vi "Lab Panel V5.12.vi"() -> ()   [LabVIEW 2013] (continued)
                            n1494 = local write "DISP LAB05-2"(w2801) -> ()
                          }
                        }
                      }
                      frame False {
                      }
                    }
                  }
                }
              }
            }
          }
          frame #6 {
            # "end test & close test files"
            n1495 = local read "MAIL SETTINGS"() -> (w2807:T7)
            n1496 = Unbundle(w2807) -> ("OUT SERVER ADDRESS"=w2806:string, "FROM ACCOUNT"=w2805:string)  [unwired: 5 out]
            n1497 = stacked-sequence {
              tunnel: w2817 -> [_ _ _ _ _ _ _ _ _ _]
              tunnel: w2818 -> [_ _ _ _ _ _ _ _ _ _]
              tunnel: w2816 -> [_ _ _ _ _ _ _ _ _ _]
              tunnel: w2815 -> [_ _ _ _ _ _ _ _ _ _]
              tunnel: w2814 -> [_ _ _ _ _ _ _ _ _ _]
              tunnel: w2813 -> [_ _ _ _ _ _ _ _ _ _]
              tunnel: w2812 -> [_ _ _ _ _ _ _ _ _ _]
              tunnel: w2811 -> [_ _ _ _ _ _ _ _ _ _]
              tunnel: w2810 -> [_ _ _ _ _ _ _ _ _ _]
              tunnel: w2809 -> [_ _ _ _ _ _ _ _ _ _]
              tunnel: w2806 -> [w2822 w2874 w2922 w2969 w3016 w3063 w3110 w3157 w3204 w3251]
              tunnel: w2805 -> [w2821 w2873 w2921 w2968 w3015 w3062 w3109 w3156 w3203 w3250]
              tunnel: "Mail Test File To:" -> [w2820 w2872 w2920 w2967 w3014 w3061 w3108 w3155 w3202 w3249]
              tunnel: "Mail Test Fail" -> [w2819 w2871 w2919 w2966 w3013 w3060 w3107 w3154 w3201 w3248]
              frame #0 {
                # "LAB01-1"
                n1498 = local read "DISP LAB01-1"() -> (w2826:T4)
                n1499 = local read "run lab01-1"() -> (w2823:bool)
                n1500 = local read "TDMS LAB01-1"() -> (w2824:refnum<k34>)
                n1501 = Unbundle(w2826) -> ("CYCLE"=w2827:dbl, "STATUS"=w2825:string)  [unwired: 1 out]
                n1502 = case shown="True" w2823 {
                  tunnel: w2827 -> [_ w2833]
                  tunnel: w2826 -> [_ w2835]
                  tunnel: w2825 -> [_ w2832]
                  tunnel: w2824 -> [_ w2834]
                  tunnel: w2822 -> [_ w2831]
                  tunnel: w2821 -> [_ w2830]
                  tunnel: w2820 -> [_ w2829]
                  tunnel: w2819 -> [_ w2828]
                  frame False {
                  }
                  frame True {
                    n1503 = Not Equal?(x=w2832, y="RUN") -> (x != y?=w2836:bool)
                    n1504 = Greater?(x=w2833, y=2.0) -> (0:w2838:bool)
                    n1505 = And(x=w2838, y=w2836) -> (x .and. y?=w2837:bool)
                    n1506 = case shown="True" w2837 {
                      tunnel: w2835 -> [_ w2848]
                      tunnel: w2834 -> [_ w2847]
                      tunnel: w2833 -> [_ w2846]
                      tunnel: w2832 -> [_ w2845]
                      tunnel: w2831 -> [_ w2844]
                      tunnel: w2830 -> [_ w2843]
                      tunnel: w2829 -> [_ w2842]
                      tunnel: w2828 -> [_ w2841]
                      frame False {
                      }
                      frame True {
                        n1507 = stacked-sequence {
                          tunnel: w2848 -> [w2852 _ _]
                          tunnel: w2847 -> [_ w2854 _]
                          tunnel: w2846 -> [_ _ _]
                          tunnel: w2845 -> [_ _ w2860]
                          tunnel: w2844 -> [_ _ w2859]
                          tunnel: w2843 -> [_ _ w2858]
                          tunnel: w2842 -> [_ _ w2857]
                          tunnel: w2841 -> [_ _ w2856]
                          frame #0 {
                            w2849 = FALSE
                            n1508 = local write "mail control"("END") -> ()
                            n1509 = Bundle(cluster=w2852) -> (w2851:T4)  [unwired: 3 in]
                            n1510 = local write "DISP LAB01-1"(w2851) -> ()
                            n1511 = local write "O/I  LAB01-1"(w2849) -> ()
                            n1512 = local write "run lab01-1"(w2849) -> ()
                            n1513 = local write "RUN LAB01-1"(w2849) -> ()
                          }
                          frame #1 {
                            n1514 = TDMS Close(11:w2854) -> (0:w2853:errorcluster)  [unwired: 1 in, 1 out]
                            n1515 = local write "data file error"(w2853) -> ()
                          }
                          frame #2 {
                            n1516 = stacked-sequence {
                              tunnel: "LAB01-1" -> [w2862 w2864 _]
                              tunnel: w2860 -> [_ w2870 _]
                              tunnel: w2859 -> [_ w2869 _]
                              tunnel: w2858 -> [_ w2868 _]
                              tunnel: w2857 -> [_ w2867 _]
                              tunnel: w2856 -> [_ w2866 _]
                              frame #0 {
                                n1517 = call "sub vi - defrag tdms v1.vi"("panel id"=w2862) -> ("error out"=w2861:errorcluster)  [unwired: 10 in]
                                n1518 = local write "data file error"(w2861) -> ()
                              }
                              frame #1 {
                                n1519 = Bundle("STATUS"=w2870, "OUT SERVER ADDRESS"=w2869, "FROM ACCOUNT"=w2868, "Mail Test File To:"=w2867, "Mail Test Fail"=w2866) -> (w2863:T25)  [unwired: 1 in]
                                n1520 = call "Save data file (pass-fail) v5.vi"("Input Cluster"=w2863, "panel id"=w2864) -> ("network file save error"=w2865:errorcluster)  [unwired: 8 in, 1 out]
                                n1521 = local write "data file error"(w2865) -> ()
                              }
                              frame #2 {
                              }
                            }
                          }
                        }
                      }
                    }
                  }
                }
              }
              frame #1 {
                # "LAB01-2"
                n1522 = local read "run lab01-2"() -> (w2875:bool)
                n1523 = case shown="True" w2875 {
                  tunnel: w2874 -> [_ w2879]
                  tunnel: w2873 -> [_ w2878]
                  tunnel: w2872 -> [_ w2877]
                  tunnel: w2871 -> [_ w2876]
                  frame False {
                  }
                  frame True {
                    n1524 = local read "DISP LAB01-2"() -> (w2887:T4)
                    n1525 = local read "TDMS LAB01-2"() -> (w2886:refnum<k34>)
                    n1526 = Unbundle(w2887) -> ("CYCLE"=w2881:dbl, "STATUS"=w2880:string)  [unwired: 1 out]
                    n1527 = Not Equal?(x=w2880, y="RUN") -> (x != y?=w2883:bool)
                    n1528 = Greater?(x=w2881, y=2.0) -> (0:w2884:bool)
                    n1529 = And(x=w2884, y=w2883) -> (x .and. y?=w2882:bool)
                    n1530 = case shown="True" w2882 {
                      tunnel: w2887 -> [_ w2896]
                      tunnel: w2886 -> [_ w2895]
                      tunnel: w2881 -> [_ w2894]
                      tunnel: w2880 -> [_ w2893]
                      tunnel: w2879 -> [_ w2892]
                      tunnel: w2878 -> [_ w2891]
                      tunnel: w2877 -> [_ w2890]
                      tunnel: w2876 -> [_ w2889]
                      frame False {
                      }
                      frame True {
                        n1531 = stacked-sequence {
                          tunnel: w2896 -> [w2899 _ _]
                          tunnel: w2895 -> [_ w2901 _]
                          tunnel: w2894 -> [_ _ _]
                          tunnel: w2893 -> [_ _ w2907]
                          tunnel: w2892 -> [_ _ w2906]
                          tunnel: w2891 -> [_ _ w2905]
                          tunnel: w2890 -> [_ _ w2904]
                          tunnel: w2889 -> [_ _ w2903]
                          frame #0 {
                            w2897 = FALSE
                            n1532 = local write "mail control"("END") -> ()
                            n1533 = Bundle(cluster=w2899) -> (w2900:T4)  [unwired: 3 in]
                            n1534 = local write "RUN LAB01-2"(w2897) -> ()
                            n1535 = local write "run lab01-2"(w2897) -> ()
                            n1536 = local write "O/I  LAB01-2"(w2897) -> ()
                            n1537 = local write "DISP LAB01-2"(w2900) -> ()
                          }
                          frame #1 {
                            n1538 = TDMS Close(11:w2901) -> (0:w2902:errorcluster)  [unwired: 1 in, 1 out]
                            n1539 = local write "data file error"(w2902) -> ()
                          }
                          frame #2 {
                            n1540 = stacked-sequence {
                              tunnel: "LAB01-2" -> [w2910 w2911]
                              tunnel: w2907 -> [_ w2916]
                              tunnel: w2906 -> [_ w2915]
                              tunnel: w2905 -> [_ w2914]
                              tunnel: w2904 -> [_ w2913]
                              tunnel: w2903 -> [_ w2912]
                              frame #0 {
                                n1541 = call "sub vi - defrag tdms v1.vi"("panel id"=w2910) -> ("error out"=w2909:errorcluster)  [unwired: 10 in]
                                n1542 = local write "data file error"(w2909) -> ()
                              }
                              frame #1 {
                                n1543 = Bundle("STATUS"=w2916, "OUT SERVER ADDRESS"=w2915, "FROM ACCOUNT"=w2914, "Mail Test File To:"=w2913, "Mail Test Fail"=w2912) -> (w2918:T25)  [unwired: 1 in]
                                n1544 = call "Save data file (pass-fail) v5.vi"("Input Cluster"=w2918, "panel id"=w2911) -> ("network file save error"=w2917:errorcluster)  [unwired: 8 in, 1 out]
                                n1545 = local write "data file error"(w2917) -> ()
                              }
                            }
                          }
                        }
                      }
                    }
                  }
                }
              }
              frame #2 {
                # "LAB02-1"
                n1546 = local read "run lab02-1"() -> (w2923:bool)
                n1547 = case shown="True" w2923 {
                  tunnel: w2922 -> [_ w2927]
                  tunnel: w2921 -> [_ w2926]
                  tunnel: w2920 -> [_ w2925]
                  tunnel: w2919 -> [_ w2924]
                  frame False {
                  }
                  frame True {
                    n1548 = local read "DISP LAB02-1"() -> (w2935:T4)
                    n1549 = Unbundle(w2935) -> ("CYCLE"=w2931:dbl, "STATUS"=w2928:string)  [unwired: 1 out]
                    n1550 = local read "TDMS LAB02-1"() -> (w2934:refnum<k34>)
                    n1551 = Not Equal?(x=w2928, y="RUN") -> (x != y?=w2930:bool)
                    n1552 = Greater?(x=w2931, y=2.0) -> (0:w2932:bool)
                    n1553 = And(x=w2932, y=w2930) -> (x .and. y?=w2929:bool)
                    n1554 = case shown="True" w2929 {
                      tunnel: w2935 -> [_ w2943]
                      tunnel: w2934 -> [_ w2942]
                      tunnel: w2928 -> [_ w2941]
                      tunnel: w2927 -> [_ w2940]
                      tunnel: w2926 -> [_ w2939]
                      tunnel: w2925 -> [_ w2938]
                      tunnel: w2924 -> [_ w2937]
                      frame False {
                      }
                      frame True {
                        n1555 = stacked-sequence {
                          tunnel: w2943 -> [w2946 _ _]
                          tunnel: w2942 -> [_ w2948 _]
                          tunnel: w2941 -> [_ _ w2954]
                          tunnel: w2940 -> [_ _ w2953]
                          tunnel: w2939 -> [_ _ w2952]
                          tunnel: w2938 -> [_ _ w2951]
                          tunnel: w2937 -> [_ _ w2950]
                          frame #0 {
                            w2944 = FALSE
                            n1556 = local write "mail control"("END") -> ()
                            n1557 = Bundle(cluster=w2946) -> (w2947:T4)  [unwired: 3 in]
                            n1558 = local write "O/I  LAB02-1"(w2944) -> ()
                            n1559 = local write "RUN LAB02-1"(w2944) -> ()
                            n1560 = local write "run lab02-1"(w2944) -> ()
                            n1561 = local write "DISP LAB02-1"(w2947) -> ()
                          }
                          frame #1 {
                            n1562 = TDMS Close(11:w2948) -> (0:w2949:errorcluster)  [unwired: 1 in, 1 out]
                            n1563 = local write "data file error"(w2949) -> ()
                          }
                          frame #2 {
                            n1564 = stacked-sequence {
                              tunnel: "LAB02-1" -> [w2957 w2964]
                              tunnel: w2954 -> [_ w2962]
                              tunnel: w2953 -> [_ w2961]
                              tunnel: w2952 -> [_ w2960]
                              tunnel: w2951 -> [_ w2959]
                              tunnel: w2950 -> [_ w2958]
                              frame #0 {
                                n1565 = call "sub vi - defrag tdms v1.vi"("panel id"=w2957) -> ("error out"=w2956:errorcluster)  [unwired: 10 in]
                                n1566 = local write "data file error"(w2956) -> ()
                              }
                              frame #1 {
                                n1567 = Bundle("STATUS"=w2962, "OUT SERVER ADDRESS"=w2961, "FROM ACCOUNT"=w2960, "Mail Test File To:"=w2959, "Mail Test Fail"=w2958) -> (w2963:T25)  [unwired: 1 in]
                                n1568 = call "Save data file (pass-fail) v5.vi"("Input Cluster"=w2963, "panel id"=w2964) -> ("network file save error"=w2965:errorcluster)  [unwired: 8 in, 1 out]
                                n1569 = local write "data file error"(w2965) -> ()
                              }
                            }
                          }
                        }
                      }
                    }
                  }
                }
              }
              frame #3 {
                # "LAB02-2"
                n1570 = local read "run lab02-2"() -> (w2970:bool)
                n1571 = case shown="True" w2970 {
                  tunnel: w2969 -> [_ w2974]
                  tunnel: w2968 -> [_ w2973]
                  tunnel: w2967 -> [_ w2972]
                  tunnel: w2966 -> [_ w2971]
                  frame False {
                  }
                  frame True {
                    n1572 = local read "DISP LAB02-2"() -> (w2982:T4)
                    n1573 = local read "TDMS LAB02-2"() -> (w2981:refnum<k34>)
                    n1574 = Unbundle(w2982) -> ("CYCLE"=w2978:dbl, "STATUS"=w2975:string)  [unwired: 1 out]
                    n1575 = Not Equal?(x=w2975, y="RUN") -> (x != y?=w2977:bool)
                    n1576 = Greater?(x=w2978, y=2.0) -> (0:w2979:bool)
                    n1577 = And(x=w2979, y=w2977) -> (x .and. y?=w2976:bool)
                    n1578 = case shown="True" w2976 {
                      tunnel: w2982 -> [_ w2990]
                      tunnel: w2981 -> [_ w2989]
                      tunnel: w2975 -> [_ w2988]
                      tunnel: w2974 -> [_ w2987]
                      tunnel: w2973 -> [_ w2986]
                      tunnel: w2972 -> [_ w2985]
                      tunnel: w2971 -> [_ w2984]
                      frame False {
                      }
                      frame True {
                        n1579 = stacked-sequence {
                          tunnel: w2990 -> [w2993 _ _]
                          tunnel: w2989 -> [_ w2995 _]
                          tunnel: w2988 -> [_ _ w3001]
                          tunnel: w2987 -> [_ _ w3000]
                          tunnel: w2986 -> [_ _ w2999]
                          tunnel: w2985 -> [_ _ w2998]
                          tunnel: w2984 -> [_ _ w2997]
                          frame #0 {
                            w2991 = FALSE
                            n1580 = local write "mail control"("END") -> ()
                            n1581 = Bundle(cluster=w2993) -> (w2994:T4)  [unwired: 3 in]
                            n1582 = local write "O/I  LAB02-2"(w2991) -> ()
                            n1583 = local write "run lab02-2"(w2991) -> ()
                            n1584 = local write "RUN LAB02-2"(w2991) -> ()
                            n1585 = local write "DISP LAB02-2"(w2994) -> ()
                          }
                          frame #1 {
                            n1586 = TDMS Close(11:w2995) -> (0:w2996:errorcluster)  [unwired: 1 in, 1 out]
                            n1587 = local write "data file error"(w2996) -> ()
                          }
                          frame #2 {
                            n1588 = stacked-sequence {
                              tunnel: "LAB02-2" -> [w3004 w3010]
                              tunnel: w3001 -> [_ w3009]
                              tunnel: w3000 -> [_ w3008]
                              tunnel: w2999 -> [_ w3007]
                              tunnel: w2998 -> [_ w3006]
                              tunnel: w2997 -> [_ w3005]
                              frame #0 {
                                n1589 = call "sub vi - defrag tdms v1.vi"("panel id"=w3004) -> ("error out"=w3003:errorcluster)  [unwired: 10 in]
                                n1590 = local write "data file error"(w3003) -> ()
                              }
                              frame #1 {
                                n1591 = Bundle("STATUS"=w3009, "OUT SERVER ADDRESS"=w3008, "FROM ACCOUNT"=w3007, "Mail Test File To:"=w3006, "Mail Test Fail"=w3005) -> (w3012:T25)  [unwired: 1 in]
                                n1592 = call "Save data file (pass-fail) v5.vi"("Input Cluster"=w3012, "panel id"=w3010) -> ("network file save error"=w3011:errorcluster)  [unwired: 8 in, 1 out]
                                n1593 = local write "data file error"(w3011) -> ()
                              }
                            }
                          }
                        }
                      }
                    }
                  }
                }
              }
              frame #4 {
                # "LAB03-1"
                n1594 = local read "run lab03-1"() -> (w3017:bool)
                n1595 = case shown="True" w3017 {
                  tunnel: w3016 -> [_ w3021]
                  tunnel: w3015 -> [_ w3020]
                  tunnel: w3014 -> [_ w3019]
                  tunnel: w3013 -> [_ w3018]
                  frame False {
                  }
                  frame True {
                    n1596 = local read "DISP LAB03-1"() -> (w3029:T4)
                    n1597 = local read "TDMS LAB03-1"() -> (w3028:refnum<k34>)
                    n1598 = Unbundle(w3029) -> ("CYCLE"=w3025:dbl, "STATUS"=w3022:string)  [unwired: 1 out]
                    n1599 = Not Equal?(x=w3022, y="RUN") -> (x != y?=w3024:bool)
                    n1600 = Greater?(x=w3025, y=2.0) -> (0:w3026:bool)
                    n1601 = And(x=w3026, y=w3024) -> (x .and. y?=w3023:bool)
                    n1602 = case shown="True" w3023 {
                      tunnel: w3029 -> [_ w3037]
                      tunnel: w3028 -> [_ w3036]
                      tunnel: w3022 -> [_ w3035]
                      tunnel: w3021 -> [_ w3034]
                      tunnel: w3020 -> [_ w3033]
                      tunnel: w3019 -> [_ w3032]
                      tunnel: w3018 -> [_ w3031]
                      frame False {
                      }
                      frame True {
                        n1603 = stacked-sequence {
                          tunnel: w3037 -> [w3040 _ _]
                          tunnel: w3036 -> [_ w3042 _]
                          tunnel: w3035 -> [_ _ w3048]
                          tunnel: w3034 -> [_ _ w3047]
                          tunnel: w3033 -> [_ _ w3046]
                          tunnel: w3032 -> [_ _ w3045]
                          tunnel: w3031 -> [_ _ w3044]
                          frame #0 {
                            w3038 = FALSE
                            n1604 = local write "mail control"("END") -> ()
                            n1605 = Bundle(cluster=w3040) -> (w3041:T4)  [unwired: 3 in]
                            n1606 = local write "O/I  LAB03-1"(w3038) -> ()
                            n1607 = local write "run lab03-1"(w3038) -> ()
                            n1608 = local write "RUN LAB03-1"(w3038) -> ()
                            n1609 = local write "DISP LAB03-1"(w3041) -> ()
                          }
                          frame #1 {
                            n1610 = TDMS Close(11:w3042) -> (0:w3043:errorcluster)  [unwired: 1 in, 1 out]
                            n1611 = local write "data file error"(w3043) -> ()
                          }
                          frame #2 {
                            n1612 = stacked-sequence {
                              tunnel: "LAB03-1" -> [w3051 w3057]
                              tunnel: w3048 -> [_ w3056]
                              tunnel: w3047 -> [_ w3055]
                              tunnel: w3046 -> [_ w3054]
                              tunnel: w3045 -> [_ w3053]
                              tunnel: w3044 -> [_ w3052]
                              frame #0 {
                                n1613 = call "sub vi - defrag tdms v1.vi"("panel id"=w3051) -> ("error out"=w3050:errorcluster)  [unwired: 10 in]
                                n1614 = local write "data file error"(w3050) -> ()
                              }
                              frame #1 {
                                n1615 = Bundle("STATUS"=w3056, "OUT SERVER ADDRESS"=w3055, "FROM ACCOUNT"=w3054, "Mail Test File To:"=w3053, "Mail Test Fail"=w3052) -> (w3059:T25)  [unwired: 1 in]
                                n1616 = call "Save data file (pass-fail) v5.vi"("Input Cluster"=w3059, "panel id"=w3057) -> ("network file save error"=w3058:errorcluster)  [unwired: 8 in, 1 out]
                                n1617 = local write "data file error"(w3058) -> ()
                              }
                            }
                          }
                        }
                      }
                    }
                  }
                }
              }
              frame #5 {
                # "LAB03-2"
                n1618 = local read "run lab03-2"() -> (w3064:bool)
                n1619 = case shown="True" w3064 {
                  tunnel: w3063 -> [_ w3068]
                  tunnel: w3062 -> [_ w3067]
                  tunnel: w3061 -> [_ w3066]
                  tunnel: w3060 -> [_ w3065]
                  frame False {
                  }
                  frame True {
                    n1620 = local read "DISP LAB03-2"() -> (w3076:T4)
                    n1621 = Unbundle(w3076) -> ("CYCLE"=w3072:dbl, "STATUS"=w3069:string)  [unwired: 1 out]
                    n1622 = local read "TDMS LAB03-2"() -> (w3075:refnum<k34>)
                    n1623 = Not Equal?(x=w3069, y="RUN") -> (x != y?=w3071:bool)
                    n1624 = Greater?(x=w3072, y=2.0) -> (0:w3073:bool)
                    n1625 = And(x=w3073, y=w3071) -> (x .and. y?=w3070:bool)
                    n1626 = case shown="True" w3070 {
                      tunnel: w3076 -> [_ w3084]
                      tunnel: w3075 -> [_ w3083]
                      tunnel: w3069 -> [_ w3082]
                      tunnel: w3068 -> [_ w3081]
                      tunnel: w3067 -> [_ w3080]
                      tunnel: w3066 -> [_ w3079]
                      tunnel: w3065 -> [_ w3078]
                      frame False {
                      }
                      frame True {
                        n1627 = stacked-sequence {
                          tunnel: w3084 -> [w3087 _ _]
                          tunnel: w3083 -> [_ w3089 _]
                          tunnel: w3082 -> [_ _ w3095]
                          tunnel: w3081 -> [_ _ w3094]
                          tunnel: w3080 -> [_ _ w3093]
                          tunnel: w3079 -> [_ _ w3092]
                          tunnel: w3078 -> [_ _ w3091]
                          frame #0 {
                            w3085 = FALSE
                            n1628 = local write "mail control"("END") -> ()
                            n1629 = Bundle(cluster=w3087) -> (w3088:T4)  [unwired: 3 in]
                            n1630 = local write "RUN LAB03-2"(w3085) -> ()
                            n1631 = local write "O/I  LAB03-2"(w3085) -> ()
                            n1632 = local write "DISP LAB03-2"(w3088) -> ()
                            n1633 = local write "run lab03-2"(w3085) -> ()
                          }
                          frame #1 {
                            n1634 = TDMS Close(11:w3089) -> (0:w3090:errorcluster)  [unwired: 1 in, 1 out]
                            n1635 = local write "data file error"(w3090) -> ()
                          }
                          frame #2 {
                            n1636 = stacked-sequence {
                              tunnel: "LAB03-2" -> [w3098 w3099]
                              tunnel: w3095 -> [_ w3104]
                              tunnel: w3094 -> [_ w3103]
                              tunnel: w3093 -> [_ w3102]
                              tunnel: w3092 -> [_ w3101]
                              tunnel: w3091 -> [_ w3100]
                              frame #0 {
                                n1637 = call "sub vi - defrag tdms v1.vi"("panel id"=w3098) -> ("error out"=w3097:errorcluster)  [unwired: 10 in]
                                n1638 = local write "data file error"(w3097) -> ()
                              }
                              frame #1 {
                                n1639 = Bundle("STATUS"=w3104, "OUT SERVER ADDRESS"=w3103, "FROM ACCOUNT"=w3102, "Mail Test File To:"=w3101, "Mail Test Fail"=w3100) -> (w3106:T25)  [unwired: 1 in]
                                n1640 = call "Save data file (pass-fail) v5.vi"("Input Cluster"=w3106, "panel id"=w3099) -> ("network file save error"=w3105:errorcluster)  [unwired: 8 in, 1 out]
                                n1641 = local write "data file error"(w3105) -> ()
                              }
                            }
                          }
                        }
                      }
                    }
                  }
                }
              }
              frame #6 {
                # "LAB04-1"
                n1642 = local read "run lab04-1"() -> (w3111:bool)
                n1643 = case shown="True" w3111 {
                  tunnel: w3110 -> [_ w3115]
                  tunnel: w3109 -> [_ w3114]
                  tunnel: w3108 -> [_ w3113]
                  tunnel: w3107 -> [_ w3112]
                  frame False {
                  }
                  frame True {
                    n1644 = local read "DISP LAB04-1"() -> (w3123:T4)
                    n1645 = Unbundle(w3123) -> ("CYCLE"=w3119:dbl, "STATUS"=w3116:string)  [unwired: 1 out]
                    n1646 = local read "TDMS LAB04-1"() -> (w3122:refnum<k34>)
                    n1647 = Not Equal?(x=w3116, y="RUN") -> (x != y?=w3118:bool)
                    n1648 = Greater?(x=w3119, y=2.0) -> (0:w3120:bool)
                    n1649 = And(x=w3120, y=w3118) -> (x .and. y?=w3117:bool)
                    n1650 = case shown="True" w3117 {
                      tunnel: w3123 -> [_ w3131]
                      tunnel: w3122 -> [_ w3130]
                      tunnel: w3116 -> [_ w3129]
                      tunnel: w3115 -> [_ w3128]
                      tunnel: w3114 -> [_ w3127]
                      tunnel: w3113 -> [_ w3126]
                      tunnel: w3112 -> [_ w3125]
                      frame False {
                      }
                      frame True {
                        n1651 = stacked-sequence {
                          tunnel: w3131 -> [w3134 _ _]
                          tunnel: w3130 -> [_ w3136 _]
                          tunnel: w3129 -> [_ _ w3142]
                          tunnel: w3128 -> [_ _ w3141]
                          tunnel: w3127 -> [_ _ w3140]
                          tunnel: w3126 -> [_ _ w3139]
                          tunnel: w3125 -> [_ _ w3138]
                          frame #0 {
                            w3132 = FALSE
                            n1652 = local write "mail control"("END") -> ()
                            n1653 = Bundle(cluster=w3134) -> (w3135:T4)  [unwired: 3 in]
                            n1654 = local write "RUN LAB04-1"(w3132) -> ()
                            n1655 = local write "O/I  LAB04-1"(w3132) -> ()
                            n1656 = local write "run lab04-1"(w3132) -> ()
                            n1657 = local write "DISP LAB04-1"(w3135) -> ()
                          }
                          frame #1 {
                            n1658 = TDMS Close(11:w3136) -> (0:w3137:errorcluster)  [unwired: 1 in, 1 out]
                            n1659 = local write "data file error"(w3137) -> ()
                          }
                          frame #2 {
                            n1660 = stacked-sequence {
                              tunnel: "LAB04-1" -> [w3145 w3146]
                              tunnel: w3142 -> [_ w3151]
                              tunnel: w3141 -> [_ w3150]
                              tunnel: w3140 -> [_ w3149]
                              tunnel: w3139 -> [_ w3148]
                              tunnel: w3138 -> [_ w3147]
                              frame #0 {
                                n1661 = call "sub vi - defrag tdms v1.vi"("panel id"=w3145) -> ("error out"=w3144:errorcluster)  [unwired: 10 in]
                                n1662 = local write "data file error"(w3144) -> ()
                              }
                              frame #1 {
                                n1663 = Bundle("STATUS"=w3151, "OUT SERVER ADDRESS"=w3150, "FROM ACCOUNT"=w3149, "Mail Test File To:"=w3148, "Mail Test Fail"=w3147) -> (w3153:T25)  [unwired: 1 in]
                                n1664 = call "Save data file (pass-fail) v5.vi"("Input Cluster"=w3153, "panel id"=w3146) -> ("network file save error"=w3152:errorcluster)  [unwired: 8 in, 1 out]
                                n1665 = local write "data file error"(w3152) -> ()
                              }
                            }
                          }
                        }
                      }
                    }
                  }
                }
              }
              frame #7 {
                # "LAB04-2"
                n1666 = local read "run lab04-2"() -> (w3158:bool)
                n1667 = case shown="True" w3158 {
                  tunnel: w3157 -> [_ w3162]
                  tunnel: w3156 -> [_ w3161]
                  tunnel: w3155 -> [_ w3160]
                  tunnel: w3154 -> [_ w3159]
                  frame False {
                  }
                  frame True {
                    n1668 = local read "DISP LAB04-2"() -> (w3170:T4)
                    n1669 = Unbundle(w3170) -> ("CYCLE"=w3166:dbl, "STATUS"=w3163:string)  [unwired: 1 out]
                    n1670 = Not Equal?(x=w3163, y="RUN") -> (x != y?=w3165:bool)
                    n1671 = local read "TDMS LAB04-2"() -> (w3169:refnum<k34>)
                    n1672 = Greater?(x=w3166, y=2.0) -> (0:w3167:bool)
                    n1673 = And(x=w3167, y=w3165) -> (x .and. y?=w3164:bool)
                    n1674 = case shown="True" w3164 {
                      tunnel: w3170 -> [_ w3178]
                      tunnel: w3169 -> [_ w3177]
                      tunnel: w3163 -> [_ w3176]
                      tunnel: w3162 -> [_ w3175]
                      tunnel: w3161 -> [_ w3174]
                      tunnel: w3160 -> [_ w3173]
                      tunnel: w3159 -> [_ w3172]
                      frame False {
                      }
                      frame True {
                        n1675 = stacked-sequence {
                          tunnel: w3178 -> [w3181 _ _]
                          tunnel: w3177 -> [_ w3183 _]
                          tunnel: w3176 -> [_ _ w3189]
                          tunnel: w3175 -> [_ _ w3188]
                          tunnel: w3174 -> [_ _ w3187]
                          tunnel: w3173 -> [_ _ w3186]
                          tunnel: w3172 -> [_ _ w3185]
                          frame #0 {
                            w3179 = FALSE
                            n1676 = local write "mail control"("END") -> ()
                            n1677 = Bundle(cluster=w3181) -> (w3182:T4)  [unwired: 3 in]
                            n1678 = local write "O/I  LAB04-2"(w3179) -> ()
                            n1679 = local write "RUN LAB04-2"(w3179) -> ()
                            n1680 = local write "run lab04-2"(w3179) -> ()
                            n1681 = local write "DISP LAB04-2"(w3182) -> ()
                          }
                          frame #1 {
                            n1682 = TDMS Close(11:w3183) -> (0:w3184:errorcluster)  [unwired: 1 in, 1 out]
                            n1683 = local write "data file error"(w3184) -> ()
                          }
                          frame #2 {
                            n1684 = stacked-sequence {
                              tunnel: "LAB04-2" -> [w3192 w3193]
                              tunnel: w3189 -> [_ w3198]
                              tunnel: w3188 -> [_ w3197]
                              tunnel: w3187 -> [_ w3196]
                              tunnel: w3186 -> [_ w3195]
                              tunnel: w3185 -> [_ w3194]
                              frame #0 {
                                n1685 = call "sub vi - defrag tdms v1.vi"("panel id"=w3192) -> ("error out"=w3191:errorcluster)  [unwired: 10 in]
                                n1686 = local write "data file error"(w3191) -> ()
                              }
                              frame #1 {
                                n1687 = Bundle("STATUS"=w3198, "OUT SERVER ADDRESS"=w3197, "FROM ACCOUNT"=w3196, "Mail Test File To:"=w3195, "Mail Test Fail"=w3194) -> (w3200:T25)  [unwired: 1 in]
                                n1688 = call "Save data file (pass-fail) v5.vi"("Input Cluster"=w3200, "panel id"=w3193) -> ("network file save error"=w3199:errorcluster)  [unwired: 8 in, 1 out]
                                n1689 = local write "data file error"(w3199) -> ()
                              }
                            }
                          }
                        }
                      }
                    }
                  }
                }
              }
              frame #8 {
                # "LAB05-1"
                n1690 = local read "run lab05-1"() -> (w3205:bool)
                n1691 = case shown="True" w3205 {
                  tunnel: w3204 -> [_ w3209]
                  tunnel: w3203 -> [_ w3208]
                  tunnel: w3202 -> [_ w3207]
                  tunnel: w3201 -> [_ w3206]
                  frame False {
                  }
                  frame True {
                    n1692 = local read "DISP LAB05-1"() -> (w3217:T4)
                    n1693 = Unbundle(w3217) -> ("CYCLE"=w3213:dbl, "STATUS"=w3210:string)  [unwired: 1 out]
                    n1694 = Not Equal?(x=w3210, y="RUN") -> (x != y?=w3212:bool)
                    n1695 = local read "TDMS LAB05-1"() -> (w3216:refnum<k34>)
                    n1696 = Greater?(x=w3213, y=2.0) -> (0:w3214:bool)
                    n1697 = And(x=w3214, y=w3212) -> (x .and. y?=w3211:bool)
                    n1698 = case shown="True" w3211 {
                      tunnel: w3217 -> [_ w3225]
                      tunnel: w3216 -> [_ w3224]
                      tunnel: w3210 -> [_ w3223]
                      tunnel: w3209 -> [_ w3222]
                      tunnel: w3208 -> [_ w3221]
                      tunnel: w3207 -> [_ w3220]
                      tunnel: w3206 -> [_ w3219]
                      frame False {
                      }
                      frame True {
                        n1699 = stacked-sequence {
                          tunnel: w3225 -> [w3228 _ _]
                          tunnel: w3224 -> [_ w3230 _]
                          tunnel: w3223 -> [_ _ w3236]
                          tunnel: w3222 -> [_ _ w3235]
                          tunnel: w3221 -> [_ _ w3234]
                          tunnel: w3220 -> [_ _ w3233]
                          tunnel: w3219 -> [_ _ w3232]
                          frame #0 {
                            w3226 = FALSE
                            n1700 = local write "mail control"("END") -> ()
                            n1701 = Bundle(cluster=w3228) -> (w3229:T4)  [unwired: 3 in]
                            n1702 = local write "O/I  LAB05-1"(w3226) -> ()
                            n1703 = local write "RUN LAB05-1"(w3226) -> ()
                            n1704 = local write "run lab05-1"(w3226) -> ()
                            n1705 = local write "DISP LAB05-1"(w3229) -> ()
                          }
                          frame #1 {
                            n1706 = TDMS Close(11:w3230) -> (0:w3231:errorcluster)  [unwired: 1 in, 1 out]
                            n1707 = local write "data file error"(w3231) -> ()
                          }
                          frame #2 {
                            n1708 = stacked-sequence {
                              tunnel: "LAB05-1" -> [w3239 w3245]
                              tunnel: w3236 -> [_ w3244]
                              tunnel: w3235 -> [_ w3243]
                              tunnel: w3234 -> [_ w3242]
                              tunnel: w3233 -> [_ w3241]
                              tunnel: w3232 -> [_ w3240]
                              frame #0 {
                                n1709 = call "sub vi - defrag tdms v1.vi"("panel id"=w3239) -> ("error out"=w3238:errorcluster)  [unwired: 10 in]
                                n1710 = local write "data file error"(w3238) -> ()
                              }
                              frame #1 {
                                n1711 = Bundle("STATUS"=w3244, "OUT SERVER ADDRESS"=w3243, "FROM ACCOUNT"=w3242, "Mail Test File To:"=w3241, "Mail Test Fail"=w3240) -> (w3247:T25)  [unwired: 1 in]
                                n1712 = call "Save data file (pass-fail) v5.vi"("Input Cluster"=w3247, "panel id"=w3245) -> ("network file save error"=w3246:errorcluster)  [unwired: 8 in, 1 out]
                                n1713 = local write "data file error"(w3246) -> ()
                              }
                            }
                          }
                        }
                      }
                    }
                  }
                }
              }
              frame #9 {
                # "LAB05-2"
                n1714 = local read "run lab05-2"() -> (w3252:bool)
                n1715 = case shown="True" w3252 {
                  tunnel: w3251 -> [_ w3256]
                  tunnel: w3250 -> [_ w3255]
                  tunnel: w3249 -> [_ w3254]
                  tunnel: w3248 -> [_ w3253]
                  frame False {
                  }
                  frame True {
                    n1716 = local read "DISP LAB05-2"() -> (w3264:T4)
                    n1717 = Unbundle(w3264) -> ("CYCLE"=w3260:dbl, "STATUS"=w3257:string)  [unwired: 1 out]
                    n1718 = Not Equal?(x=w3257, y="RUN") -> (x != y?=w3259:bool)
                    n1719 = local read "TDMS LAB05-2"() -> (w3263:refnum<k34>)
                    n1720 = Greater?(x=w3260, y=2.0) -> (0:w3261:bool)
                    n1721 = And(x=w3261, y=w3259) -> (x .and. y?=w3258:bool)
                    n1722 = case shown="True" w3258 {
                      tunnel: w3264 -> [_ w3272]
                      tunnel: w3263 -> [_ w3271]
                      tunnel: w3257 -> [_ w3270]
                      tunnel: w3256 -> [_ w3269]
                      tunnel: w3255 -> [_ w3268]
                      tunnel: w3254 -> [_ w3267]
                      tunnel: w3253 -> [_ w3266]
                      frame False {
                      }
                      frame True {
                        n1723 = stacked-sequence {
                          tunnel: w3272 -> [w3275 _ _]
                          tunnel: w3271 -> [_ w3277 _]
                          tunnel: w3270 -> [_ _ w3283]
                          tunnel: w3269 -> [_ _ w3282]
                          tunnel: w3268 -> [_ _ w3281]
                          tunnel: w3267 -> [_ _ w3280]
                          tunnel: w3266 -> [_ _ w3279]
                          frame #0 {
                            w3273 = FALSE
                            n1724 = local write "mail control"("END") -> ()
                            n1725 = Bundle(cluster=w3275) -> (w3276:T4)  [unwired: 3 in]
                            n1726 = local write "RUN LAB05-2"(w3273) -> ()
                            n1727 = local write "O/I  LAB05-2"(w3273) -> ()
                            n1728 = local write "run lab05-2"(w3273) -> ()
                            n1729 = local write "DISP LAB05-2"(w3276) -> ()
                          }
                          frame #1 {
                            n1730 = TDMS Close(11:w3277) -> (0:w3278:errorcluster)  [unwired: 1 in, 1 out]
                            n1731 = local write "data file error"(w3278) -> ()
                          }
                          frame #2 {
                            n1732 = stacked-sequence {
                              tunnel: "LAB05-2" -> [w3286 w3292]
                              tunnel: w3283 -> [_ w3291]
                              tunnel: w3282 -> [_ w3290]
                              tunnel: w3281 -> [_ w3289]
                              tunnel: w3280 -> [_ w3288]
                              tunnel: w3279 -> [_ w3287]
                              frame #0 {
                                n1733 = call "sub vi - defrag tdms v1.vi"("panel id"=w3286) -> ("error out"=w3285:errorcluster)  [unwired: 10 in]
                                n1734 = local write "data file error"(w3285) -> ()
                              }
                              frame #1 {
                                n1735 = Bundle("STATUS"=w3291, "OUT SERVER ADDRESS"=w3290, "FROM ACCOUNT"=w3289, "Mail Test File To:"=w3288, "Mail Test Fail"=w3287) -> (w3294:T25)  [unwired: 1 in]
                                n1736 = call "Save data file (pass-fail) v5.vi"("Input Cluster"=w3294, "panel id"=w3292) -> ("network file save error"=w3293:errorcluster)  [unwired: 8 in, 1 out]
                                n1737 = local write "data file error"(w3293) -> ()
                              }
                            }
                          }
                        }
                      }
                    }
                  }
                }
              }
            }
            n1738 = local read "Network Directory"() -> (w2808:path)
            n1739 = global write "Global 1.vi" "Network Drive"(w2808) -> ()
          }
          frame #7 {
            # "disable functions"
            n1740 = stacked-sequence {
              tunnel: w3304 -> [w3318 _ w3375]
              tunnel: w3303 -> [w3313 _ w3374]
              tunnel: w3302 -> [w3312 _ w3373]
              tunnel: w3301 -> [w3310 _ w3372]
              tunnel: w3300 -> [w3311 _ w3371]
              tunnel: w3299 -> [_ w3335 w3370]
              tunnel: w3298 -> [_ w3336 w3369]
              tunnel: w3297 -> [_ w3337 w3368]
              tunnel: w3296 -> [_ w3338 w3367]
              tunnel: w3295 -> [_ w3339 w3366]
              frame #0 {
                n1741 = Select(t=2, s=w3310, f=0) -> (s? t:f=w3306:i32)
                n1742 = Select(t=2, s=w3312, f=0) -> (s? t:f=w3307:i32)
                n1743 = Select(t=2, s=w3311, f=0) -> (s? t:f=w3305:i32)
                n1744 = Select(t=2, s=w3318, f=0) -> (s? t:f=w3309:i32)
                n1745 = Select(t=2, s=w3313, f=0) -> (s? t:f=w3308:i32)
                n1746 = property on="SELECT LAB02-2" class="RadioBtnsControl (strict)"("DisabledEnum"=w3306) -> ()  [unwired: 2 in, 2 out]
                n1747 = property on="SELECT LAB02-1" class="RadioBtnsControl (strict)"("DisabledEnum"=w3307) -> ()  [unwired: 2 in, 2 out]
                n1748 = property on="SELECT LAB03-1" class="RadioBtnsControl (strict)"("DisabledEnum"=w3305) -> ()  [unwired: 2 in, 2 out]
                n1749 = property on="SELECT LAB01-1" class="RadioBtnsControl (strict)"("DisabledEnum"=w3309) -> ()  [unwired: 2 in, 2 out]
                n1750 = property on="SELECT LAB01-2" class="RadioBtnsControl (strict)"("DisabledEnum"=w3308) -> ()  [unwired: 2 in, 2 out]
                n1751 = Not(x=w3318) -> (.not. x?=w3319:bool)
                n1752 = property on="RESULT LAB01-1" class="Bool (strict)"("Visible"=w3319) -> ()  [unwired: 2 in, 2 out]
                n1753 = Not(x=w3313) -> (.not. x?=w3317:bool)
                n1754 = Not(x=w3312) -> (.not. x?=w3316:bool)
                n1755 = Not(x=w3310) -> (.not. x?=w3315:bool)
                n1756 = property on="RESULT LAB01-2" class="Bool (strict)"("Visible"=w3317) -> ()  [unwired: 2 in, 2 out]
                n1757 = Not(x=w3311) -> (.not. x?=w3314:bool)
                n1758 = property on="RESULT LAB02-1" class="Bool (strict)"("Visible"=w3316) -> ()  [unwired: 2 in, 2 out]
                n1759 = property on="RESULT LAB02-2" class="Bool (strict)"("Visible"=w3315) -> ()  [unwired: 2 in, 2 out]
                n1760 = property on="RESULT LAB03-1" class="Bool (strict)"("Visible"=w3314) -> ()  [unwired: 2 in, 2 out]
                n1761 = property on="SET LAB01-1" class="Clust (strict)"("DisabledEnum"=w3309) -> ()  [unwired: 2 in, 2 out]
                n1762 = property on="SET LAB01-2" class="Clust (strict)"("DisabledEnum"=w3308) -> ()  [unwired: 2 in, 2 out]
                n1763 = property on="SET LAB02-1" class="Clust (strict)"("DisabledEnum"=w3307) -> ()  [unwired: 2 in, 2 out]
                n1764 = property on="SET LAB02-2" class="Clust (strict)"("DisabledEnum"=w3306) -> ()  [unwired: 2 in, 2 out]
                n1765 = property on="SET LAB03-1" class="Clust (strict)"("DisabledEnum"=w3305) -> ()  [unwired: 2 in, 2 out]
                n1766 = property on="O/I  LAB01-1" class="Bool (strict)"("DisabledEnum"=w3309) -> ()  [unwired: 2 in, 2 out]
                n1767 = property on="O/I  LAB01-2" class="Bool (strict)"("DisabledEnum"=w3308) -> ()  [unwired: 2 in, 2 out]
                n1768 = property on="O/I  LAB02-1" class="Bool (strict)"("DisabledEnum"=w3307) -> ()  [unwired: 2 in, 2 out]
                n1769 = property on="O/I  LAB02-2" class="Bool (strict)"("DisabledEnum"=w3306) -> ()  [unwired: 2 in, 2 out]
                n1770 = property on="O/I  LAB03-1" class="Bool (strict)"("DisabledEnum"=w3305) -> ()  [unwired: 2 in, 2 out]
              }
              frame #1 {
                n1771 = Select(t=2, s=w3339, f=0) -> (s? t:f=w3330:i32)
                n1772 = Select(t=2, s=w3338, f=0) -> (s? t:f=w3331:i32)
                n1773 = Select(t=2, s=w3335, f=0) -> (s? t:f=w3334:i32)
                n1774 = Select(t=2, s=w3336, f=0) -> (s? t:f=w3333:i32)
                n1775 = Select(t=2, s=w3337, f=0) -> (s? t:f=w3332:i32)
                n1776 = property on="SELECT LAB05-2" class="RadioBtnsControl (strict)"("DisabledEnum"=w3330) -> ()  [unwired: 2 in, 2 out]
                n1777 = property on="SELECT LAB05-1" class="RadioBtnsControl (strict)"("DisabledEnum"=w3331) -> ()  [unwired: 2 in, 2 out]
                n1778 = property on="SELECT LAB03-2" class="RadioBtnsControl (strict)"("DisabledEnum"=w3334) -> ()  [unwired: 2 in, 2 out]
                n1779 = property on="SELECT LAB04-1" class="RadioBtnsControl (strict)"("DisabledEnum"=w3333) -> ()  [unwired: 2 in, 2 out]
                n1780 = property on="SELECT LAB04-2" class="RadioBtnsControl (strict)"("DisabledEnum"=w3332) -> ()  [unwired: 2 in, 2 out]
                n1781 = property on="SET LAB05-2" class="Clust (strict)"("DisabledEnum"=w3330) -> ()  [unwired: 2 in, 2 out]
                n1782 = property on="SET LAB05-1" class="Clust (strict)"("DisabledEnum"=w3331) -> ()  [unwired: 2 in, 2 out]
                n1783 = property on="SET LAB03-2" class="Clust (strict)"("DisabledEnum"=w3334) -> ()  [unwired: 2 in, 2 out]
                n1784 = property on="SET LAB04-1" class="Clust (strict)"("DisabledEnum"=w3333) -> ()  [unwired: 2 in, 2 out]
                n1785 = property on="SET LAB04-2" class="Clust (strict)"("DisabledEnum"=w3332) -> ()  [unwired: 2 in, 2 out]
                n1786 = property on="O/I  LAB05-2" class="Bool (strict)"("DisabledEnum"=w3330) -> ()  [unwired: 2 in, 2 out]
                n1787 = property on="O/I  LAB05-1" class="Bool (strict)"("DisabledEnum"=w3331) -> ()  [unwired: 2 in, 2 out]
                n1788 = property on="O/I  LAB04-1" class="Bool (strict)"("DisabledEnum"=w3333) -> ()  [unwired: 2 in, 2 out]
                n1789 = property on="O/I  LAB04-2" class="Bool (strict)"("DisabledEnum"=w3332) -> ()  [unwired: 2 in, 2 out]
                n1790 = property on="O/I  LAB03-2" class="Bool (strict)"("DisabledEnum"=w3334) -> ()  [unwired: 2 in, 2 out]
                n1791 = Not(x=w3339) -> (.not. x?=w3340:bool)
                n1792 = Not(x=w3338) -> (.not. x?=w3341:bool)
